vi "Write Stored State DVR.vi"(8 "error in (no error)":errorcluster, 10 "Stored State DVR":refnum<data-value>, 11 "Display Data in":refnum<class "Display Data.lvclass">) -> (0 "error out":errorcluster, 3 "Display Data out":refnum<class "Display Data.lvclass">)   [LabVIEW 2013, in "Display Data.lvclass"]
uses:
  Display Data.lvclass
  State data/State Data.lvclass
  Display Data.lvclass/Display Data.ctl
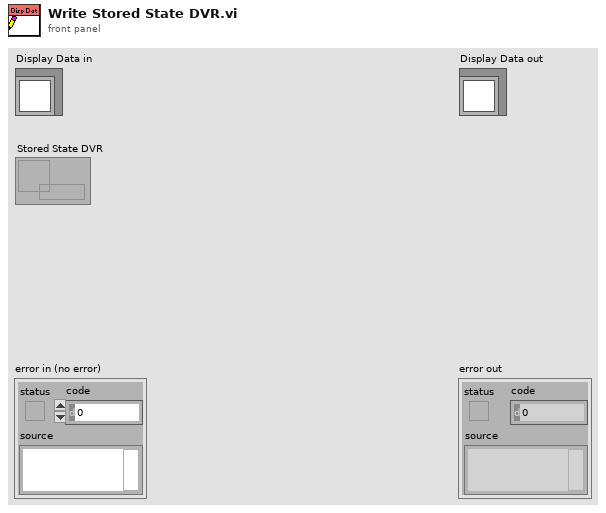
[diagram p1: front panel]
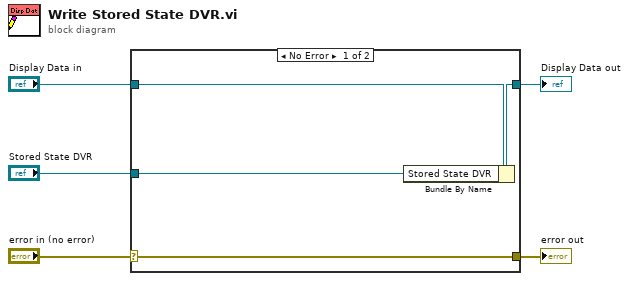
[diagram p0: block diagram]
diagram:
  n1 = case shown="No Error" "error in (no error)" {
    selector: "error in (no error)" -> [w9 w10]
    tunnel: [w9 w10] -> w4
    tunnel: [w7 w11] -> w2
    tunnel: "Display Data in" -> [w8 w11]
    tunnel: "Stored State DVR" -> [w6 _]
    frame No Error {
      n2 = Bundle By Name(cluster=w8, "Stored State DVR"=w6) -> (w7:refnum<class "Display Data.lvclass">)
    }
    frame Error {
    }
  }
  "error out" <- w4
  "Display Data out" <- w2
